vi "PramsSpeedTest.vi"() -> ()   [LabVIEW 2011]
panel:
  out "MessageTypeEnum":u32
  out "MessageLength":u32
  out "Signature":u32
  out "ACK":u32
  out "Total":u32
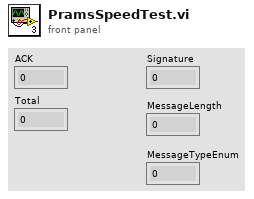
[diagram p1: front panel]
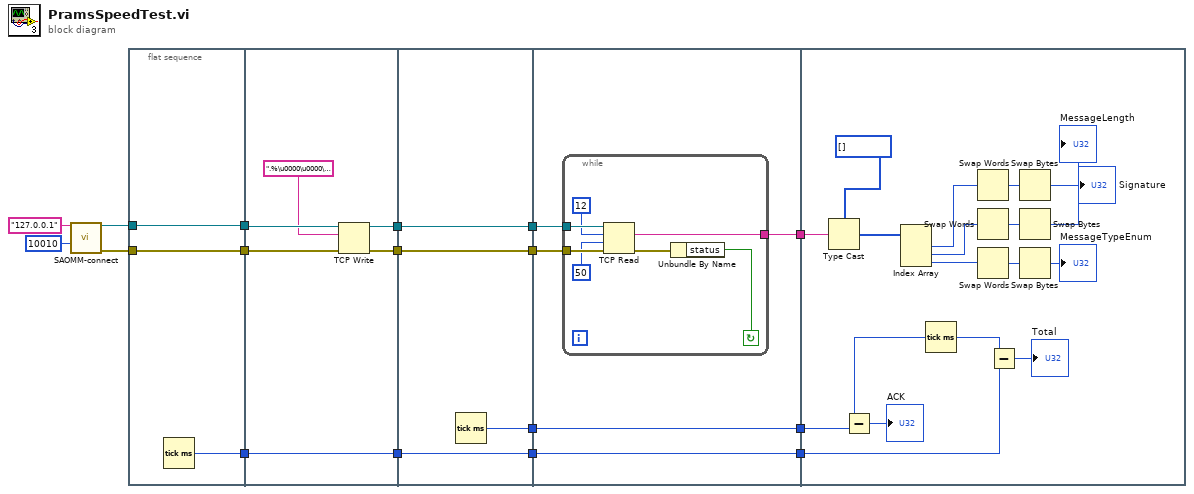
[diagram p0: block diagram]
diagram:
  n1 = call "SAOMM-connect.vi"("IP"="127.0.0.1", "Port"=u16 10010) -> ("connection ID"=w15:refnum<k5>, "Error OUT"=w14:errorcluster)  [unwired: 12 in]
  n2 = flat-sequence {
    tunnel: w14 -> [w19]
    tunnel: w15 -> [w20]
    tunnel: [w20] -> w13
    tunnel: [w19] -> w12
    tunnel: [w18] -> w3
    tunnel: w13 -> [w26]
    tunnel: w12 -> [w25]
    tunnel: [w23] -> w10
    tunnel: [w22] -> w8
    tunnel: [w21] -> w4
    tunnel: w3 -> [w21]
    tunnel: [w30] -> w11
    tunnel: w10 -> [w30]
    tunnel: [w29] -> w9
    tunnel: w8 -> [w29]
    tunnel: [w28] -> w5
    tunnel: w4 -> [w28]
    tunnel: [w27] -> w1
    tunnel: w11 -> [w35]
    tunnel: w9 -> [w34]
    tunnel: [w33] -> w7
    tunnel: [w32] -> w6
    tunnel: w5 -> [w32]
    tunnel: [w31] -> w2
    tunnel: w1 -> [w31]
    tunnel: w7 -> [w54]
    tunnel: w6 -> [w59]
    tunnel: w2 -> [w56]
    frame #0 {
      n3 = Tick Count (ms)() -> (millisecond timer value=w18:u32)
    }
    frame #1 {
      n4 = TCP Write(connection ID=w26, data in=".%\u0000\u0000\u000e\u0000\u0000\u0000V\u0004\u0000\u00002\u0000", error in (no error)=w25) -> (connection ID out=w23:refnum<k5>, error out=w22:errorcluster)  [unwired: 1 in, 1 out]
    }
    frame #2 {
      n5 = Tick Count (ms)() -> (millisecond timer value=w27:u32)
    }
    frame #3 {
      n6 = while {
        tunnel: w35 -> [w42]
        tunnel: w34 -> [w41]
        tunnel: [w36] -> w33
        stop <- w39 continue-if-true
        n7 = TCP Read(connection ID=w42, bytes to read=12, error in (no error)=w41, 9:50 ("timeout ms (25000)")) -> (data out=w36:string, error out=w40:errorcluster)  [unwired: 1 in, 1 out]
        n8 = Unbundle By Name(w40) -> ("status"=w39:bool)
      }
    }
    frame #4 {
      n9 = Type Cast(type=u32[] [], x=w54) -> (*(type *) &x=w52:u32[])
      n10 = Index Array(array=w52) -> (element #1=w46:u32, element #2=w47:u32, element #3=w48:u32)  [unwired: 3 in]
      n11 = Tick Count (ms)() -> (millisecond timer value=w55:u32)
      n12 = Subtract(x=w55, y=w56) -> (x-y=→"ACK":u32)
      n13 = Swap Words(1:w46) -> (0:w51:u32)
      n14 = Swap Words(1:w47) -> (0:w50:u32)
      n15 = Swap Words(1:w48) -> (0:w49:u32)
      n16 = Subtract(x=w55, y=w59) -> (x-y=→"Total":u32)
      n17 = Swap Bytes(anything=w51) -> (byte swapped=→"Signature":u32)
      n18 = Swap Bytes(anything=w50) -> (byte swapped=→"MessageLength":u32)
      n19 = Swap Bytes(anything=w49) -> (byte swapped=→"MessageTypeEnum":u32)
    }
  }
